vi "Save to TDMS Core.vi"(8 "Error In":errorcluster, 10 "TDMS Ref":refnum<k34>, 11 "LHW-Data in":refnum<class "LHW-Data.lvclass">) -> (0 "Error Out":errorcluster, 3 "LHW-Data out":refnum<class "LHW-Data.lvclass">)   [LabVIEW 2016, in "LHW-Data.lvlib" / "LHW-Data.lvclass"]
doc: "Save data to TDMS file."
uses:
  LHW-Data.lvclass
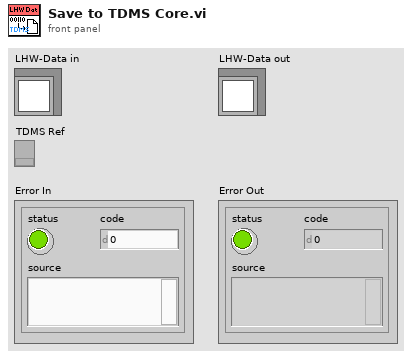
[diagram p1: front panel]
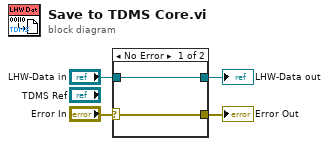
[diagram p0: block diagram]
diagram:
  n1 = case shown="No Error" "Error In" {
    selector: "Error In" -> [w5 w8]
    tunnel: [w5 w8] -> w3
    tunnel: [w6 w7] -> w1
    tunnel: "LHW-Data in" -> [w6 w7]
    frame No Error {
    }
    frame Error {
    }
  }
  "Error Out" <- w3
  "LHW-Data out" <- w1
